vi "Clear myQuake.vi"(8 "error in (no error)":errorcluster, 11 "task array In":refnum<k21>[](array[refnum])) -> (0 "error out":errorcluster)   [LabVIEW 2013]
doc: "Turns off all outputs and clears the 3 DAQmx tasks created for myQuake."
uses:
  <vilib>/DAQmx/write.llb/DAQmx Write (Digital 1D Bool NChan 1Samp 1Line).vi
  <vilib>/DAQmx/miscellaneous.llb/DAQmx Fill In Error Info.vi
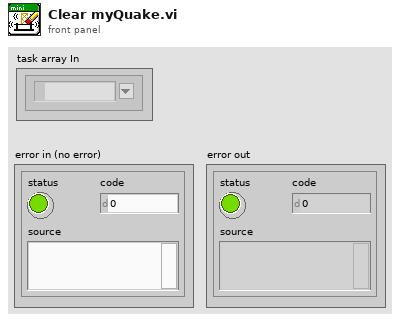
[diagram p1: front panel]
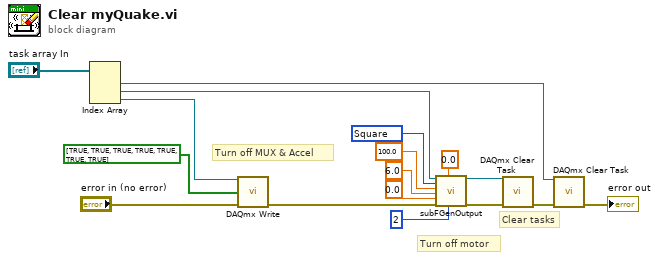
[diagram p0: block diagram]
diagram:
  w10 = 14753 items=["Sine"=14751, "Triangle"=14752, "Square"=14753, "Sawtooth"=14754] ("AO.FuncGen.Type")
  # "Clear tasks"
  # "Turn off MUX & Accel"
  # "Turn off motor"
  n1 = Index Array(array="task array In") -> (element #1=w16:refnum<k21>, element #2=w4:refnum<k21>, element #3=w15:refnum<k21>)  [unwired: 3 in]
  n2 = call-poly <vilib>:"DAQmx Write.vi"("task/channels in"=w15, "data"=bool[] [TRUE, TRUE, TRUE, TRUE, TRUE, TRUE, TRUE], "error in"="error in (no error)") -> ("error out"=w6:errorcluster)  [unwired: 10 in, 2 out]
  n3 = call <vilib>:"subFGenOutput.vi"("task in"=w4, "AO.FuncGen.Type"=w10, "Frequency"=100.0 ("frequency"), "Amplitude"=6.0 ("amplitude"), "Offset"=0.0, "error in (no error)"=w6, "square wave duty cycle (%)"=0.0, "Signal Type"=2) -> ("task out"=w8:refnum<k21>, "error out"=w7:errorcluster)  [unwired: 9 in, 1 out]
  n4 = call <vilib>:"DAQmx Clear Task.vi"("task in"=w8, "error in"=w7) -> ("error out"=w17:errorcluster)  [unwired: 13 in]
  n5 = call <vilib>:"DAQmx Clear Task.vi"("task in"=w16, "error in"=w17) -> ("error out"=→"error out":errorcluster)  [unwired: 13 in]
